vi "Pic2SubAp.vi"() -> ()   [LabVIEW 2014]
uses:
  <vilib>/picture/picture.llb/imagedata.ctl
  <vilib>/picture/picture.llb/Draw True-Color Pixmap.vi
  <vilib>/vision/NI_Vision_Development_Module.lvlib
panel:
  in  "Index":u32
  in  "SavePath":path
  in  "Angle":dbl
  in  "Overlap%":dbl
  in  "SubApPix":u32
  out "Intensity Graph":u8[][](graph)
  out "output array":u8[][](array[numeric])
  out "image data":T1
  in  "Path":path
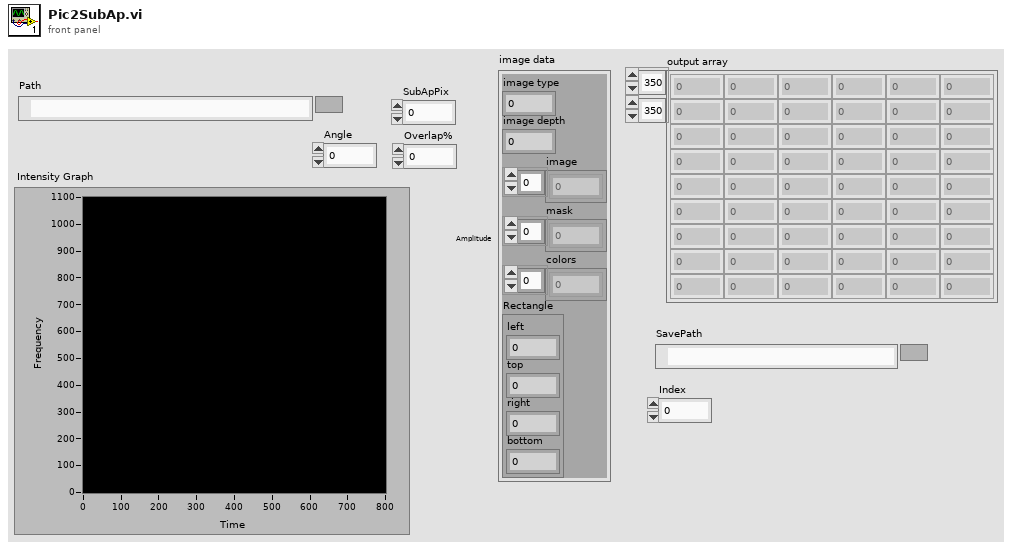
[diagram p1: front panel]
types:
  T1 = typedef "imagedata.ctl" = cluster{"image type":i32, "image depth":i32, "image":u8[], "mask":u8[], "colors":u32[], "Rectangle":cluster{"left":i16, "top":i16, "right":i16, "bottom":i16}}
  T2 = typedef "Image Type" = u32
  T3 = typedef "IMAQ Image.ctl" = refnum<image>
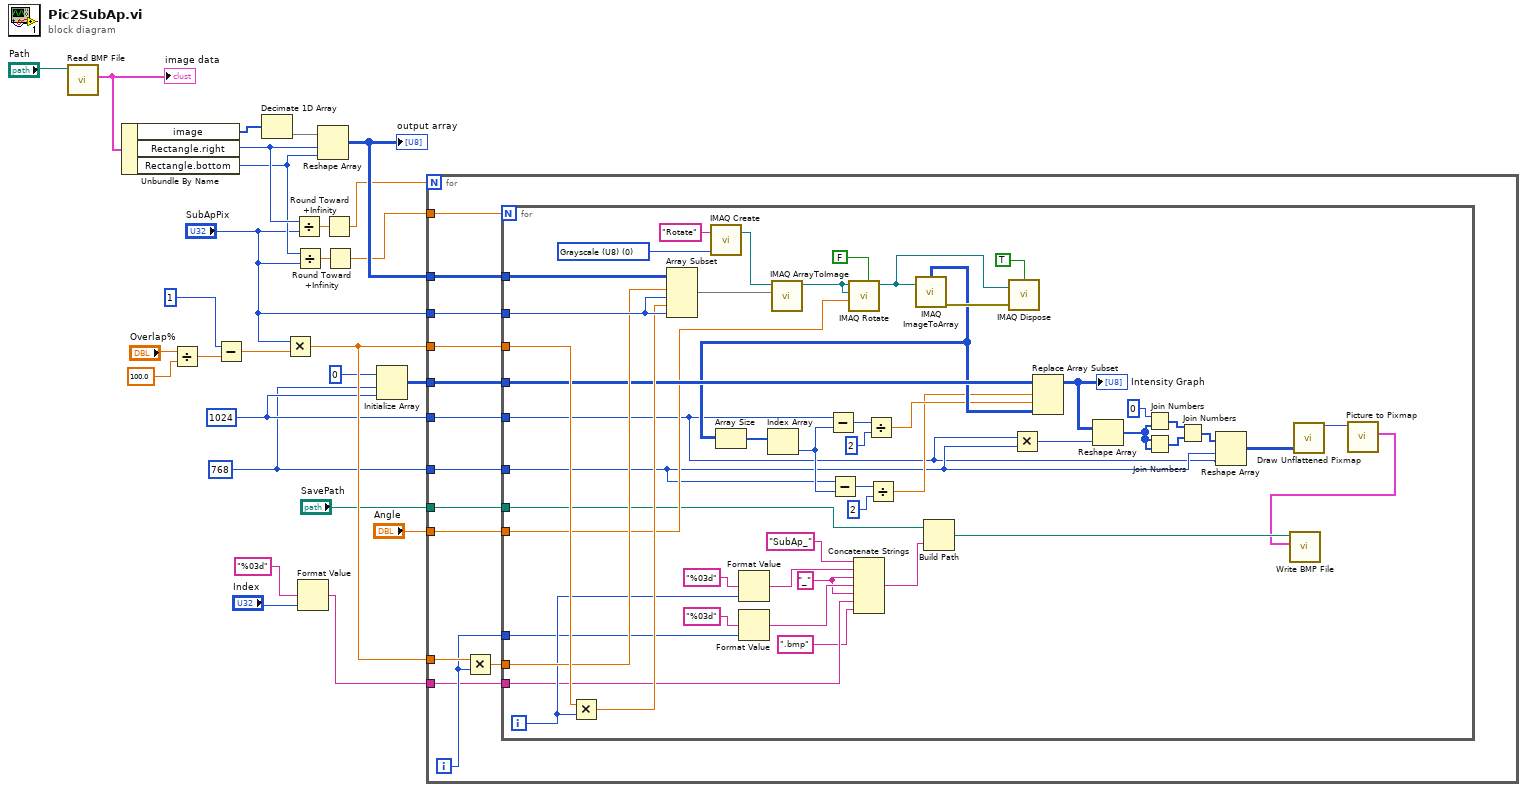
[diagram p0: block diagram]
diagram:
  w5 = 768
  w6 = 1024
  n1 = call <vilib>:"Read BMP File.vi"("path to BMP file"="Path") -> ("image data"=w26:T1)  [unwired: 8 in, 2 out]
  "image data" <- w26
  n2 = Unbundle By Name(w26) -> ("image"=w25:u8[], "Rectangle.right"=w22:i16, "Rectangle.bottom"=w19:i16)
  n3 = Divide(x="Overlap%", y=100.0) -> (x/y=w13:dbl)
  n4 = Subtract(x=1, y=w13) -> (x-y=w12:dbl)
  n5 = Decimate 1D Array(w25) -> (w24:u8[])  [unwired: 2 out]
  n6 = Multiply(x="SubApPix", y=w12) -> (x*y=w11:dbl)
  n7 = Divide(x=w22, y="SubApPix") -> (x/y=w21:dbl)
  n8 = Divide(x=w19, y="SubApPix") -> (x/y=w20:dbl)
  n9 = Format Value(format string="%03d", value (0)="Index") -> (output string=w2:string)  [unwired: 1 in]
  n10 = Reshape Array(w24, w22, w19) -> (w23:u8[][])
  "output array" <- w23
  n11 = Round Toward +Infinity(x=w21) -> (ceil(x): smallest int >= x=w18:dbl)
  n12 = Round Toward +Infinity(x=w20) -> (ceil(x): smallest int >= x=w17:dbl)
  n13 = Initialize Array(u8 0, w5, w6) -> (w8:u8[][])
  n14 = for {
    N: w18 -> [_]
    tunnel: w23 -> [w40]
    tunnel: w17 -> [w39]
    tunnel: "SubApPix" -> [w38]
    tunnel: w11 -> [w37]
    tunnel: w11 -> [w36]
    tunnel: w8 -> [w34]
    tunnel: "Angle" -> [w33]
    tunnel: w6 -> [w32]
    tunnel: w5 -> [w31]
    tunnel: w2 -> [w29]
    tunnel: "SavePath" -> [w28]
    i -> [w30]
    n15 = Multiply(x=w36, y=w30) -> (x*y=w35:dbl)
    n16 = for {
      N: w39 -> [_]
      tunnel: w40 -> [w90]
      tunnel: w38 -> [w89]
      tunnel: w37 -> [w88]
      tunnel: w35 -> [w86]
      tunnel: w34 -> [w85]
      tunnel: w33 -> [w79]
      tunnel: w32 -> [w50]
      tunnel: w31 -> [w51]
      tunnel: w30 -> [w64]
      tunnel: w29 -> [w59]
      tunnel: w28 -> [w57]
      i -> [w66]
      w60 = "_" ("string")
      w83 = T2 0 items=["Grayscale (U8)", "Grayscale (I16)", "Grayscale (SGL)", "Complex (CSG)", "RGB (U32)", "HSL (U32)", "RGB (U64)", "Grayscale (U16)"] ("Image Type")
      n17 = Multiply(x=w88, y=w66) -> (x*y=w87:dbl)
      n18 = Array Subset(array=w90, index (row)=w86, length (row)=w89, index (col)=w87, length (col)=w89) -> (w81:u8[][])
      n19 = call "IMAQ Create"("Image Name"="Rotate", "Image Type"=w83) -> ("New Image"=w82:T3)  [unwired: 3 in, 1 out]
      n20 = Format Value(format string="%03d", value (0)=w66) -> (output string=w62:string)  [unwired: 1 in]
      n21 = Format Value(format string="%03d", value (0)=w64) -> (output string=w61:string)  [unwired: 1 in]
      n22 = call "IMAQ ArrayToImage"("Image Pixels (U8)"=w81, "Image"=w82) -> ("Image Out"=w80:T3)  [unwired: 8 in, 1 out]
      n23 = call "IMAQ Rotate"("Maintain Size"=FALSE, "Angle (degrees)"=w79, "Image Dst"=w80, "Image Src"=w80) -> ("Image Dst Out"=w77:T3)  [unwired: 6 in, 1 out]
      n24 = Concatenate Strings("SubAp_" ("string"), w62, w60, w61, w60, w59, ".bmp" ("string")) -> (w56:string)
      n25 = call "IMAQ ImageToArray"("Image"=w77) -> ("error out"=w78:errorcluster, "Image Pixels (U8)"=w68:u8[][])  [unwired: 3 in, 3 out]
      n26 = Array Size(array=w68) -> (size(s)=w70:i32[])
      n27 = Index Array(array=w70) -> (element=w69:i32)  [unwired: 1 in]
      n28 = Subtract(x=w50, y=w69) -> (x-y=w71:i32)
      n29 = Subtract(x=w51, y=w69) -> (x-y=w74:i32)
      n30 = Divide(x=w71, y=2) -> (x/y=w54:dbl)
      n31 = Divide(x=w74, y=2) -> (x/y=w53:dbl)
      n32 = Build Path(base path=w57, name or relative path=w56) -> (appended path=w48:path)
      n33 = call "IMAQ Dispose"("All Images? (No)"=TRUE, "Image"=w77, "error in (no error)"=w78) -> ()  [unwired: 3 in, 1 out]
      n34 = Multiply(x=w50, y=w51) -> (x*y=w52:i32)
      n35 = Replace Array Subset(array=w85, new element=w68, index (row)=w53, index (col)=w54) -> (w55:u8[][])
      "Intensity Graph" <- w55
      n36 = Reshape Array(w55, w52) -> (w44:u8[])
      n37 = Join Numbers(hi=u8 0, lo=w44) -> ((hi.lo)=w46:u16[])
      n38 = Join Numbers(hi=w44, lo=w44) -> ((hi.lo)=w45:u16[])
      n39 = Join Numbers(hi=w46, lo=w45) -> ((hi.lo)=w43:u32[])
      n40 = Reshape Array(w43, w51, w50) -> (w42:u32[][])
      n41 = call-poly <vilib>:"Draw Unflattened Pixmap.vi"("data (RGB format)"=w42) -> ("new picture"=w49:picture)  [unwired: 8 in]
      n42 = call <vilib>:"Picture to Pixmap.vi"("picture"=w49) -> ("image data"=w47:T1)  [unwired: 9 in, 1 out]
      n43 = call <vilib>:"Write BMP File.vi"("image data"=w47, "path to BMP file"=w48) -> ()  [unwired: 8 in, 2 out]
    }
  }
